vi "Arm Immediate with Deadband.vi"(6 "Gripper":dbl, 7 "Description":string, 8 "Command Info In":T1, 9 "Deadband Value":dbl=0.01, 10 "Shoulder Setpoint":dbl, 11 "Base Setpoint":dbl) -> (0 "Command Info Out":T1)   [LabVIEW 2017]
uses:
  <vilib>/Rock Robotics/WPI/Framework/Command Status Info.ctl
  <vilib>/Rock Robotics/WPI/Framework/Completion Status.ctl
  <vilib>/Rock Robotics/WPI/Framework/Completion Notifier.ctl
  Implementation/Arm Setpoints.ctl
  Implementation/Arm Operations.ctl
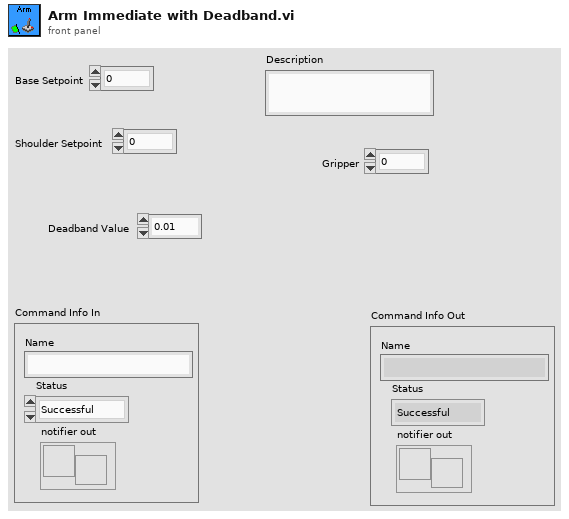
[diagram p1: front panel]
types:
  T1 = typedef "Command Status Info.ctl" = cluster{"Name":string, "Status":T2, "notifier out":T3}
  T2 = typedef "Completion Status.ctl" = enum16{"Successful", "Aborted", "Incomplete"}
  T3 = typedef "Completion Notifier.ctl" = refnum<notifier>
  T4 = typedef "Arm Setpoints.ctl" = cluster{"Operation":T5, "Duration":dbl, "Base Setpoint":dbl, "Shoulder Setpoint":dbl, "Gripper":dbl}
  T5 = typedef "Arm Operations.ctl" = enum16{"Reserve", "Read Current", "Immediate", "Close Gripper", "Open Gripper"}
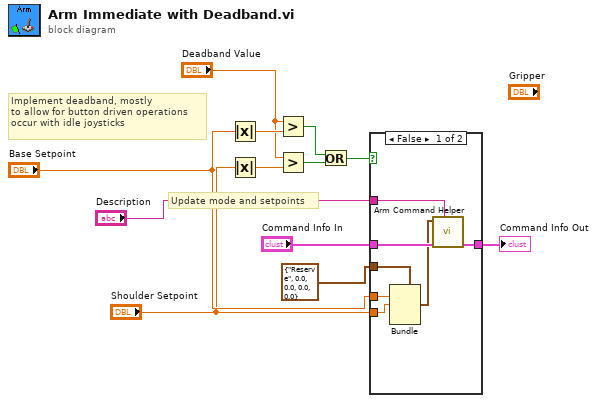
[diagram p0: block diagram]
diagram:
  # "Implement deadband, mostly\nto allow for button driven operations\noccur with idle joysticks"
  # "Update mode and setpoints"
  n1 = Absolute Value(x="Base Setpoint") -> (abs(x)=w12:dbl)
  n2 = Absolute Value(x="Shoulder Setpoint") -> (abs(x)=w5:dbl)
  n3 = Greater?(x="Deadband Value", y=w12) -> (0:w3:bool)
  n4 = Greater?(x="Deadband Value", y=w5) -> (0:w2:bool)
  n5 = Or(x=w3, y=w2) -> (x .or. y?=w4:bool)
  n6 = case shown="False" w4 {
    tunnel: "Base Setpoint" -> [w19 _]
    tunnel: T4 {"Operation"=enum."Reserve", "Duration"=0.0, "Base Setpoint"=0.0, "Shoulder Setpoint"=0.0, "Gripper"=0.0} ("SubSystem Data") -> [w18 _]
    tunnel: [w17 w20] -> w11
    tunnel: "Command Info In" -> [w16 w20]
    tunnel: "Description" -> [w14 _]
    tunnel: "Shoulder Setpoint" -> [w13 _]
    frame False {
      n7 = Bundle(cluster=w18, "Duration"=w19, "Base Setpoint"=w13) -> (w15:T4)  [unwired: 3 in]
      n8 = call "Arm Command Helper.vi"("Description"=w14, "Command Info In"=w16, "SubSystem Data"=w15) -> ("Command Info Out"=w17:T1)  [unwired: 7 in, 1 out]
    }
    frame True {
    }
  }
  "Command Info Out" <- w11
